vi "mm2time.vi"(1 "fs?":bool, 2 "Offset (mm)":dbl, 3 "distance (mm)":dbl) -> (0 "time in fs/ps seconds":dbl)   [LabVIEW 2020]
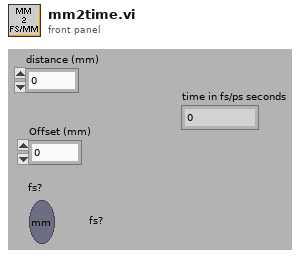
[diagram p1: front panel]
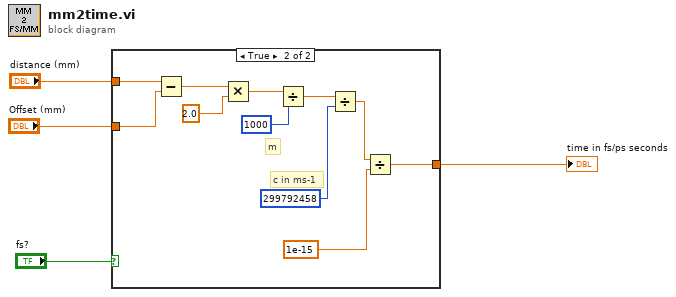
[diagram p0: block diagram]
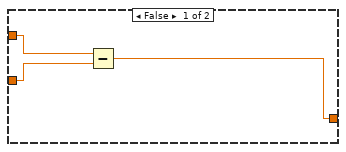
[diagram p2: hidden frame]
diagram:
  n1 = case shown="True" "fs?" {
    tunnel: [w5 w8] -> w3
    tunnel: "distance (mm)" -> [w7 w12]
    tunnel: "Offset (mm)" -> [w6 w11]
    frame False {
      n2 = Subtract(x=w7, y=w6) -> (x-y=w5:dbl)
    }
    frame True {
      # "c in ms-1"
      # "m"
      n3 = Subtract(x=w12, y=w11) -> (x-y=w13:dbl)
      n4 = Multiply(x=w13, y=2.0) -> (x*y=w15:dbl)
      n5 = Divide(x=w15, y=1000) -> (x/y=w17:dbl)
      n6 = Divide(x=w17, y=299792458) -> (x/y=w10:dbl)
      n7 = Divide(x=w10, y=1e-15) -> (x/y=w8:dbl)
    }
  }
  "time in fs/ps seconds" <- w3
